vi "LoadRecalcSave_171213.vi"(6 "Segments":bool[](array[boolean]), 8 "Time":string, 9 "Segments(s)":dbl[](array[numeric]), 10 "LoadBackPath":path, 11 "Slide in":refnum<vi>) -> (2 "ForAnalysisPath":path, 3 "ForSegmentsBMP":path)   [LabVIEW 2016]
uses:
  <vilib>/Utility/file.llb/Write Delimited Spreadsheet (string).vi
  Globaltracker.vi
panel:
  out "TTLIsActive":bool
  out "TTLOn":i32
  out "Counter":i32
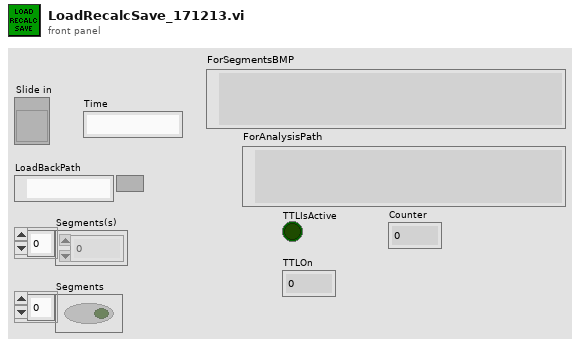
[diagram p1: front panel]
types:
  T1 = typedef "LVDateTimeRec.ctl" = cluster{"fractional second":dbl, "second":i32, "minute":i32, "hour":i32, "day of month":i32, "month":i32, "year":i32, "day of week":i32, "day of year":i32, "DST":i32}
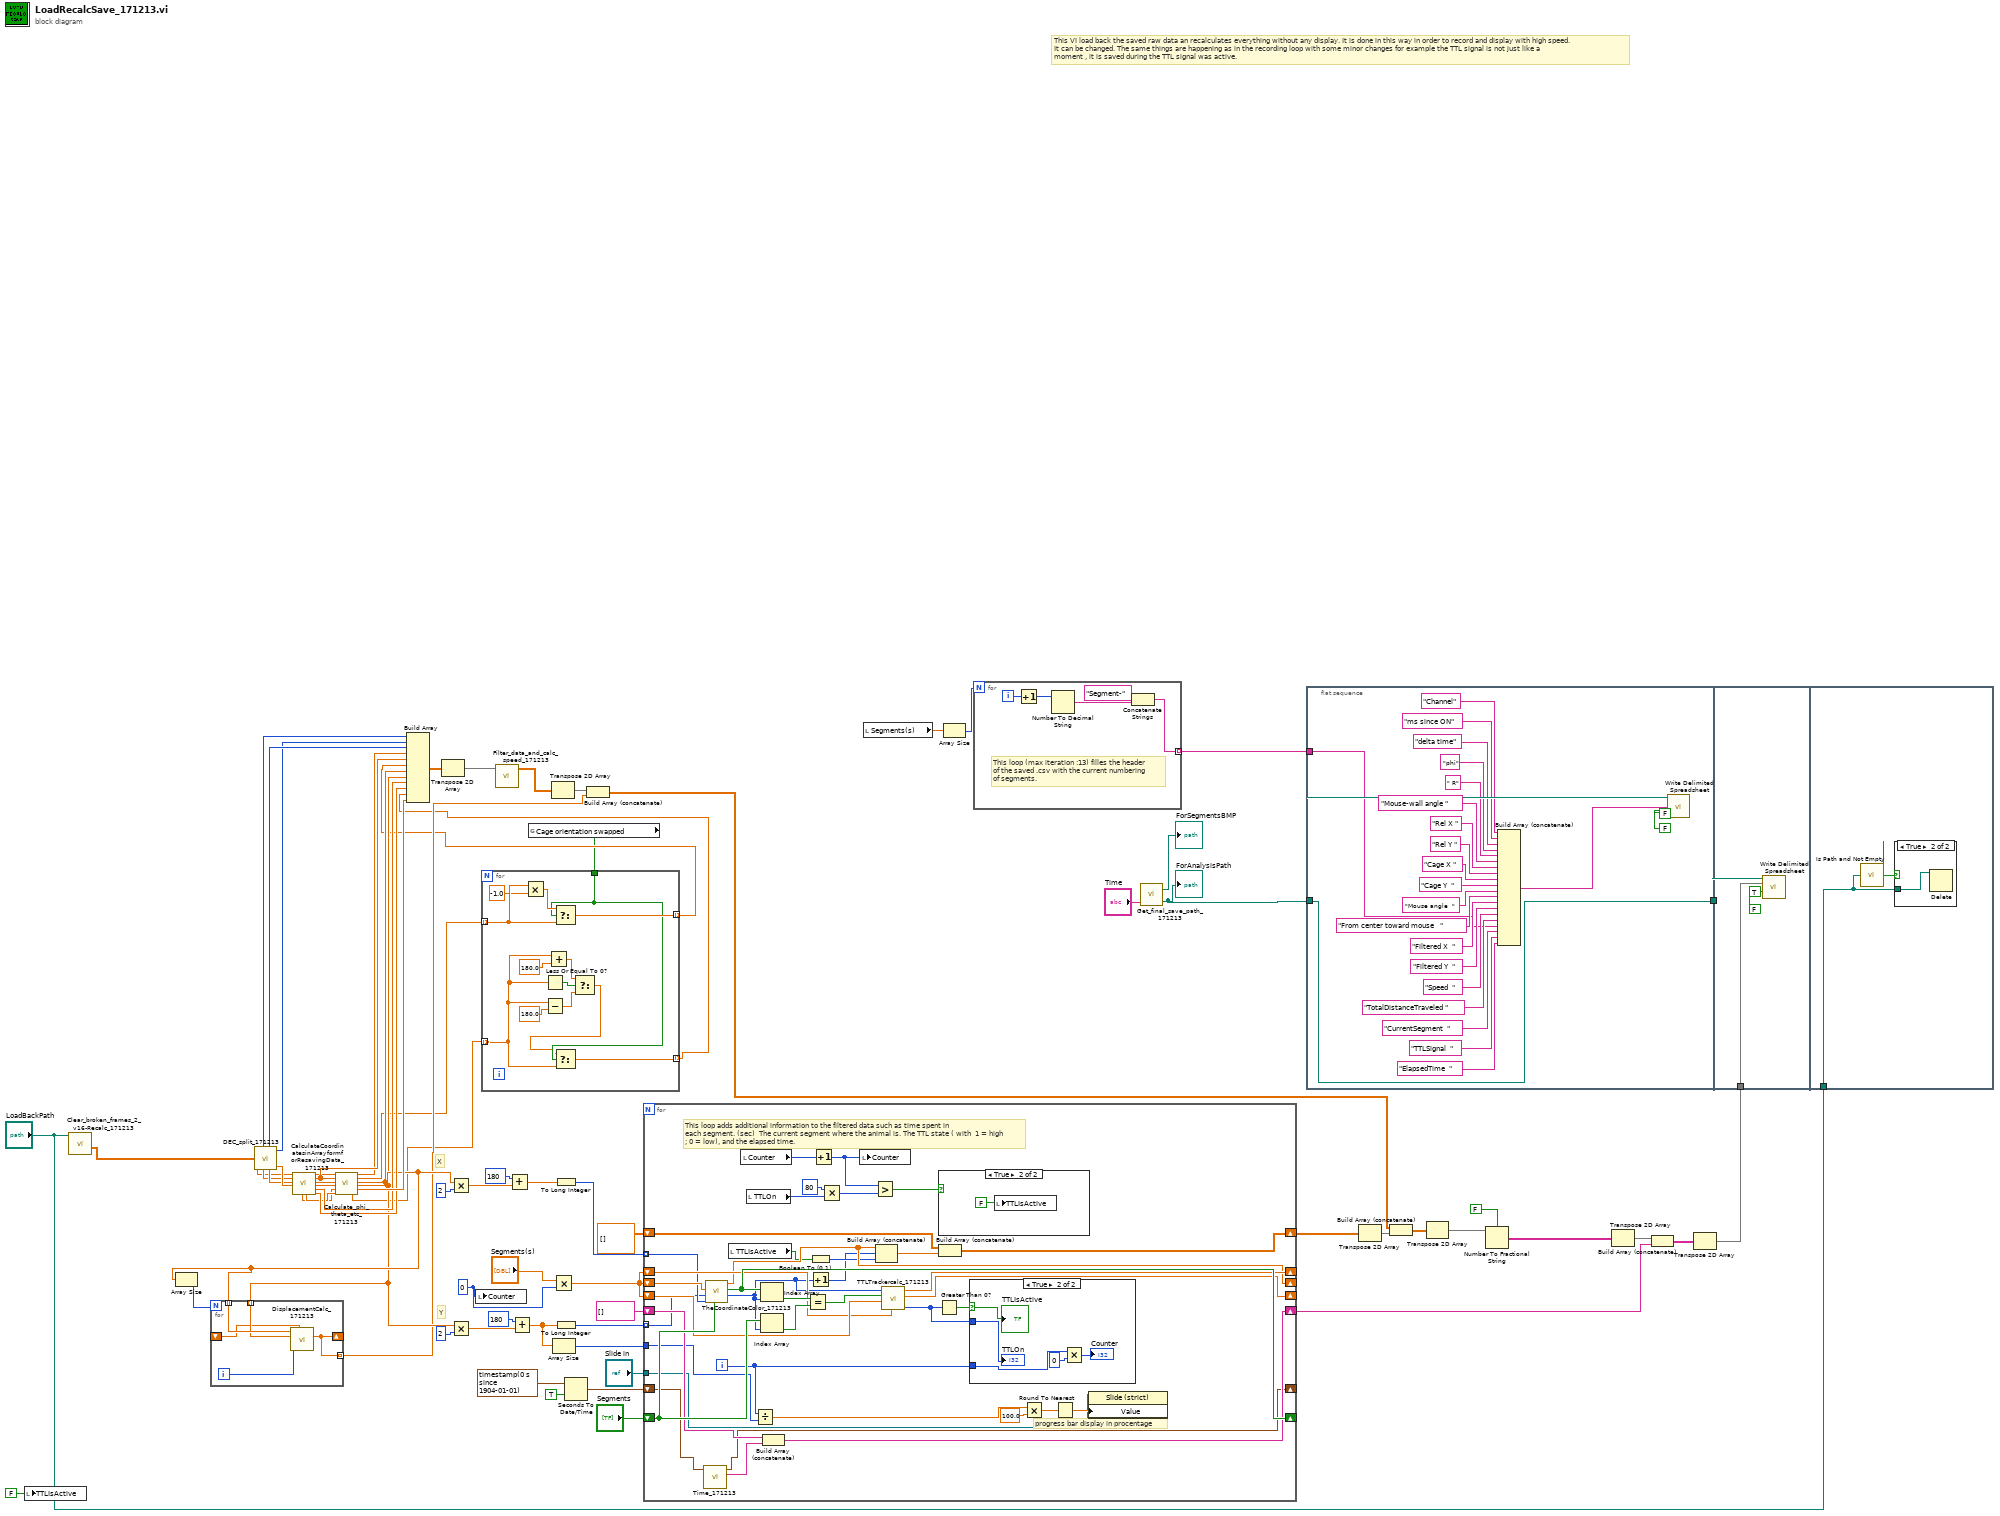
[diagram p0: block diagram]
diagram:
  w21 = 0 ("index")
  # "This VI load back the saved raw data an recalculates everything without any display. It is done in this way in order to record and display with high speed. \nIt can be changed. The same things are happening as in the recording loop with some minor changes for example the TTL signal is not just like a\nmoment , it is saved during the TTL signal was active."
  # "Y"
  # "X"
  n1 = local write "TTLIsActive"(FALSE ("TTLIsActive")) -> ()
  n2 = call "Clear_broken_frames_2_v16-Recalc_171213.vi"("file path (dialog if empty)"="LoadBackPath") -> ("Cleaned array"=w14:dbl[][])  [unwired: 8 in, 2 out]
  n3 = call "DEC_split_171213.vi"("Input DEC array"=w14) -> ("Channel"=w36:u32[], "X1"=w27:sgl[], "Y1"=w28:sgl[], "delta time"=w38:u32[], "ms since ON"=w37:u32[], "X2"=w29:sgl[], "Y2"=w30:sgl[])  [unwired: 2 in]
  n4 = call "CalculateCoordinatesinArrayformforResavingData_171213.vi"("X1"=w27, "Y1"=w28, "X2"=w29, "Y2"=w30) -> ("X1-X2"=w34:sgl[], "Y1-Y2"=w35:sgl[], "sin(a)"=w31:sgl[], "R from center"=w40:sgl[], "Mouse Xc"=w32:sgl[], "Mouse Yc"=w33:sgl[], "Cage Xc"=w41:sgl[], "Cage Yc"=w42:sgl[])  [unwired: 8 in]
  n5 = call "Calculate_phi_theta_etc_171213.vi"("sin(a)"=w31, "R from center"=w40, "Mouse Xc"=w32, "Mouse Yc"=w33, "X1-X2"=w34, "Y1-Y2"=w35) -> ("Mouse-angle"=w5:dbl[], "phi"=w39:dbl[], "Mouse-wall angle"=w4:dbl[], "Rel X"=w11:dbl[], "Rel Y"=w10:dbl[], "From center towards mouse"=w43:dbl[])  [unwired: 7 in, 1 out]
  n6 = Array Size(array=w11) -> (size(s)=w12:i32)
  n7 = for {
    N: w12 -> [_]
    tunnel: w11 -> [w76] mode=indexing
    tunnel: w10 -> [w75] mode=indexing
    shift-right: [w73] -> _
    shift-left: _ -> [w74]
    tunnel: [w73] -> w7 mode=indexing
    i -> [w77]
    n8 = call "DisplacementCalc_171213.vi"("TotalDistanceTraveledInput"=w74, "i"=w77, "Y"=w75, "X"=w76) -> ("TotalDistanceTraveledOutput"=w73:dbl)  [unwired: 6 in, 1 out]
  }
  n9 = Multiply(x=w11, y=2 ("disabled index (col)")) -> (x*y=w47:dbl[])
  n10 = Multiply(x=w10, y=2 ("disabled index (col)")) -> (x*y=w48:dbl[])
  n11 = local write "Counter"(w21) -> ()
  n12 = Add(x=180 ("disabled index (col)"), y=w47) -> (x+y=w51:dbl[])
  n13 = Add(x=180 ("disabled index (col)"), y=w48) -> (x+y=w71:dbl[])
  n14 = global read "Globaltracker.vi" "Cage orientation swapped"() -> (w2:bool)
  n15 = for {
    tunnel: w5 -> [w79] mode=indexing
    tunnel: w4 -> [w88] mode=indexing
    tunnel: [w90] -> w3 mode=indexing
    tunnel: w2 -> [w85]
    tunnel: [w86] -> w1 mode=indexing
    n16 = Multiply(x=w88, y=-1.0) -> (x*y=w89:dbl)
    n17 = Less Or Equal To 0?(x=w79) -> (x <= 0?=w84:bool)
    n18 = Subtract(x=w79, y=180.0) -> (x-y=w80:dbl)
    n19 = Add(x=w79, y=180.0) -> (x+y=w83:dbl)
    n20 = Select(t=w89, s=w85, f=w88) -> (s? t:f=w90:dbl)
    n21 = Select(t=w83, s=w84, f=w80) -> (s? t:f=w82:dbl)
    n22 = Select(t=w82, s=w85, f=w79) -> (s? t:f=w86:dbl)
  }
  n23 = Build Array ("Pack to array")(w36, w37, w38, w39, w40, w3, w11, w10, w41, w42, w1, w43) -> (w44:dbl[][])
  n24 = Transpose 2D Array(2D array=w44) -> (transposed array=w70:dbl[][])
  n25 = call "Filter_data_and_calc_speed_171213.vi"("Input array (clean)"=w70) -> ("Output"=w9:dbl[][])  [unwired: 10 in]
  n26 = Transpose 2D Array(2D array=w9) -> (transposed array=w8:dbl[][])
  n27 = Multiply(x="Segments(s)", y=w21) -> (x*y=w54:dbl[])
  n28 = Array Size(array=w71) -> (size(s)=w72:i32)
  n29 = To Long Integer(number=w51) -> (32bit integer=w52:i32[])
  n30 = To Long Integer(number=w71) -> (32bit integer=w67:i32[])
  n31 = Seconds To Date/Time(time stamp (now)=timestamp(0 s since 1904-01-01) ("current time"), to UTC (F)=TRUE) -> (date time rec=w60:T1)
  n32 = Build Array (concatenate)(w8, w7) -> (w6:dbl[][])
  n33 = for {
    tunnel: w52 -> [w96] mode=indexing
    tunnel: w67 -> [w95] mode=indexing
    shift-right: [w120] -> _
    shift-left: w54 -> [w130]
    shift-right: [w123] -> _
    shift-left: w54 -> [w124]
    shift-right: [w121] -> _
    shift-left: w54 -> [w122]
    shift-right: [w126] -> _
    shift-left: "Segments" -> [w127]
    shift-right: [w117] -> w64
    shift-left: dbl[][] [] -> [w116]
    shift-right: [w91] -> _
    shift-left: w60 -> [w93]
    shift-right: [w113] -> w66
    shift-left: string[] [] -> [w112]
    tunnel: w72 -> [w97]
    tunnel: "Slide in" -> [w107]
    i -> [w94]
    # "This loop adds additional information to the filtered data such as time spent in \neach segment. (sec)  The current segment where the animal is. The TTL state ( with  1 = high\n; 0 = low), and the elapsed time."
    # "progress bar display in procentage"
    n34 = call "Time_171213.vi"("TimeIn"=w93) -> (2:"TimeOut"=w92:string, 3:"TimeOut"=w91:T1)  [unwired: 9 in]
    n35 = call "TheCoordinateColor_171213.vi"("InputSegments"=w127, "X"=w96, "Y"=w95, "InputSegments(s)"=w130) -> ("MATCH index"=w119:i32, "Outputsegments"=w126:bool[], "OutputSegmens(s)"=w120:dbl[])  [unwired: 5 in]
    n36 = local read "TTLIsActive"() -> (w98:bool)
    n37 = local read "Counter"() -> (w105:i32)
    n38 = local read "TTLOn"() -> (w102:i32)
    n39 = Divide(x=w94, y=w97) -> (x/y=w109:dbl)
    n40 = Index Array(array=w126, index=w119) -> (element=w128:bool)
    n41 = Index Array(array=w127, index=w119) -> (element=w129:bool)
    n42 = Build Array (concatenate)(w112, w92) -> (w113:string[])
    n43 = Equal?(x=w128, y=w129) -> (x = y?=w125:bool)
    n44 = Boolean To (0,1)(Boolean=w98) -> (0, 1=w118:i16)
    n45 = Increment(x=w119) -> (x+1=w114:i32)
    n46 = Increment(x=w105) -> (x+1=w99:i32)
    n47 = Multiply(x=80, y=w102) -> (x*y=w100:i32)
    n48 = local write "Counter"(w99) -> ()
    n49 = Greater?(x=w99, y=w100) -> (0:w104:bool)
    n50 = Build Array (concatenate)(w120, w114, w118) -> (w115:dbl[])
    n51 = call "TTLTrackercalc_171213.vi"("Outside in"=w122, "Inside in"=w124, "Boolean"=w125, "MATCH index"=w119) -> ("TTLduration"=w103:i32, "Inside out"=w123:dbl[], "Outside out"=w121:dbl[])  [unwired: 5 in]
    n52 = Greater Than 0?(x=w103) -> (x > 0?=w106:bool)
    n53 = case shown="True" w104 {
      frame False {
      }
      frame True {
        n54 = local write "TTLIsActive"(FALSE ("RewardanalyzeON")) -> ()
      }
    }
    n55 = Build Array (concatenate)(w116, w115) -> (w117:dbl[][])
    n56 = case shown="True" w106 {
      selector: w106 -> [_ w132]
      tunnel: w94 -> [_ w136]
      tunnel: w103 -> [_ w133]
      frame False {
      }
      frame True {
        n57 = Multiply(x=w136, y=0) -> (x*y=→"Counter":i32)
        "TTLOn" <- w133
        "TTLIsActive" <- w132
      }
    }
    n58 = Multiply(x=w109, y=100.0) -> (x*y=w111:dbl)
    n59 = Round To Nearest(number=w111) -> (nearest integer value=w108:dbl)
    n60 = property class="Slide (strict)"(reference=w107, "Value"=w108) -> ()  [unwired: 1 in, 2 out]
  }
  n61 = local read "Segments(s)"() -> (w19:dbl[])
  n62 = Array Size(array=w19) -> (size(s)=w18:i32)
  n63 = for {
    N: w18 -> [_]
    tunnel: [w138] -> w17 mode=indexing
    i -> [w140]
    # "This loop (max iteration :13) filles the header\nof the saved .csv with the current numbering\nof segments."
    n64 = Increment(x=w140) -> (x+1=w137:i32)
    n65 = Number To Decimal String(number=w137) -> (decimal integer string=w139:string)  [unwired: 1 in]
    n66 = Concatenate Strings("Segment-", w139) -> (w138:string)
  }
  n67 = call "Get_final_save_path_171213.vi"("Time string"="Time") -> ("File output path"=w22:path, "For regions"=→"ForSegmentsBMP":path)  [unwired: 2 in]
  "ForAnalysisPath" <- w22
  n68 = flat-sequence {
    tunnel: w22 -> [w163]
    tunnel: [w163] -> w25
    tunnel: w17 -> [w145]
    tunnel: w25 -> [w169]
    tunnel: w20 -> [w168]
    tunnel: "LoadBackPath" -> [w171]
    frame #0 {
      n69 = Build Array (concatenate)("Channel", "ms since ON", "delta time", "phi", " R", "Mouse-wall angle ", "Rel X ", "Rel Y ", "Cage X ", "Cage Y  ", "Mouse angle  ", "From center toward mouse   ", "Filtered X  ", "Filtered Y  ", "Speed  ", "TotalDistanceTraveled ", w145, "CurrentSegment  ", "TTLSignal  ", "ElapsedTime  ") -> (w146:string[])
      n70 = call-poly <vilib>:"Write Delimited Spreadsheet.vi"("file path (dialog if empty)"=w163, "1D data"=w146, "append to file? (new file:F)"=FALSE, "transpose? (no:F)"=FALSE) -> ()  [unwired: 10 in, 2 out]
    }
    frame #1 {
      n71 = call-poly <vilib>:"Write Delimited Spreadsheet.vi"("file path (dialog if empty)"=w169, "2D data"=w168, "append to file? (new file:F)"=TRUE, "transpose? (no:F)"=FALSE ("append to file? (new file:F)")) -> ()  [unwired: 10 in, 2 out]
    }
    frame #2 {
      n72 = call <vilib>:"Is Path and Not Empty.vi"("path"=w171) -> ("Is Path and Not Empty?"=w170:bool)  [unwired: 4 in]
      n73 = case shown="True" w170 {
        tunnel: w171 -> [_ w172]
        frame False {
        }
        frame True {
          n74 = Delete(path (use dialog)=w172) -> ()  [unwired: 4 in, 3 out]
        }
      }
    }
  }
  n75 = Transpose 2D Array(2D array=w64) -> (transposed array=w56:dbl[][])
  n76 = Build Array (concatenate)(w6, w56) -> (w57:dbl[][])
  n77 = Transpose 2D Array(2D array=w57) -> (transposed array=w65:dbl[][])
  n78 = Number To Fractional String(use system decimal point (T)=FALSE, number=w65) -> (F-format string=w63:string[][])  [unwired: 2 in]
  n79 = Transpose 2D Array(2D array=w63) -> (transposed array=w62:string[][])
  n80 = Build Array (concatenate)(w62, w66) -> (w61:string[][])
  n81 = Transpose 2D Array(2D array=w61) -> (transposed array=w20:string[][])
